vi "Setup Refine.vi"() -> (3 "Intensity Graph Ref":refnum<vi>)   [LabVIEW 2023]
panel:
  out "Intensity Graph Setup":dbl[][](graph)
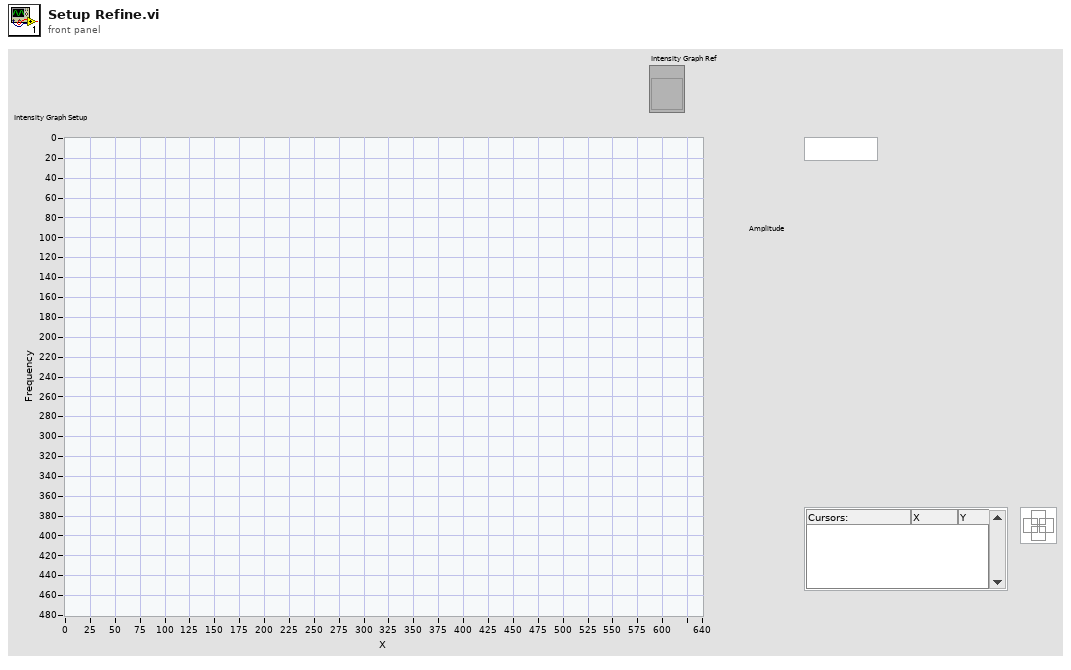
[diagram p1: front panel]
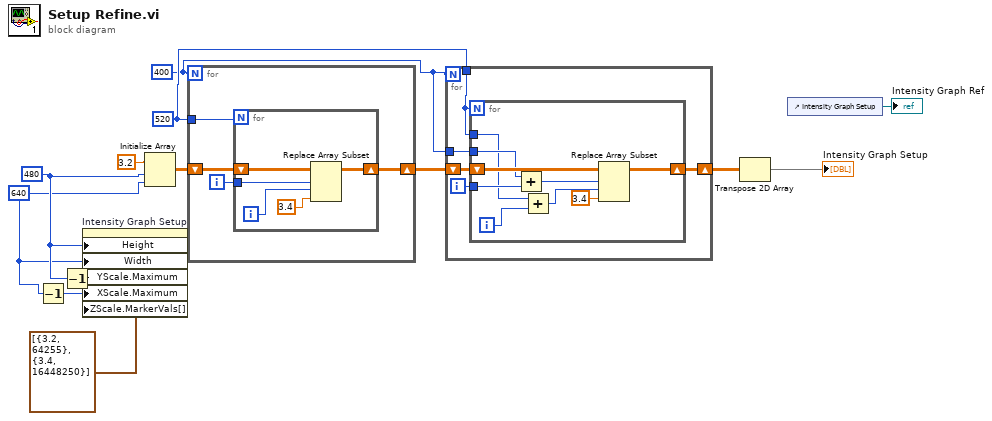
[diagram p0: block diagram]
diagram:
  w4 = 520
  w10 = 640 ("dimension size")
  w11 = 480 ("dimension size")
  w3 = 400
  n1 = Decrement(x=w10) -> (x-1=w9:i32)
  n2 = Decrement(x=w11) -> (x-1=w8:i32)
  n3 = property on="Intensity Graph Setup" class="IntGraph (strict)"("Height"=w11, "Width"=w10, "YScale.Maximum"=w8, "XScale.Maximum"=w9, "ZScale.MarkerVals[]"=cluster{dbl, u32}[] [{3.2, 64255}, {3.4, 16448250}] ("Z Scale.Marker Values[]")) -> ()  [unwired: 2 in, 2 out]
  n4 = Initialize Array(3.2 ("element"), w11, w10) -> (w12:dbl[][])
  n5 = for {
    N: w3 -> [_]
    shift-right: [w16] -> w6
    shift-left: w12 -> [w17]
    tunnel: w4 -> [w14]
    i -> [w15]
    n6 = for {
      N: w14 -> [_]
      shift-right: [w18] -> w16
      shift-left: w17 -> [w22]
      tunnel: w15 -> [w21]
      i -> [w20]
      n7 = Replace Array Subset(array=w22, new element=3.4, index (row)=w21, index (col)=w20) -> (w18:dbl[][])
    }
  }
  n8 = for {
    N: w3 -> [_]
    tunnel: w4 -> [w25]
    tunnel: w3 -> [w23]
    shift-right: [w26] -> w5
    shift-left: w6 -> [w27]
    i -> [w24]
    n9 = for {
      N: w25 -> [_]
      tunnel: w25 -> [w28]
      tunnel: w24 -> [w33]
      tunnel: w23 -> [w29]
      shift-right: [w35] -> w26
      shift-left: w27 -> [w36]
      i -> [w32]
      n10 = Add(x=w29, y=w33) -> (x+y=w34:i32)
      n11 = Add(x=w28, y=w32) -> (x+y=w31:i32)
      n12 = Replace Array Subset(array=w36, new element=3.4 ("new element/subarray"), index (row)=w34, index (col)=w31) -> (w35:dbl[][])
    }
  }
  n13 = Transpose 2D Array(2D array=w5) -> (transposed array=→"Intensity Graph Setup":dbl[][])
  n14 = control-ref of="Intensity Graph Setup"() -> (→"Intensity Graph Ref":refnum<vi>)
